vi "setRootDevice.vi"(8 "error in (no error)":errorcluster, 9 "Config in":refnum<class "IPropertyObject.lvclass">, 10 "Connection String in":string, 11 "IInstance in":refnum<class "IInstance.lvclass">) -> (0 "error out":errorcluster, 1 "Config out":refnum<class "IPropertyObject.lvclass">, 2 "Connection String out":string, 3 "IInstance out":refnum<class "IInstance.lvclass">)   [LabVIEW 2022 SP3, in "openDAQ.lvlib" / "IBaseObject.lvlib" / "IPropertyObject.lvlib" / "IComponent.lvlib" / "IFolder.lvlib" / "IDevice.lvlib" / "IInstance.lvlib" / "IInstance.lvclass"]
uses:
  <instrlib>/openDAQ/Public/Classes/IInstance/IInstance.lvclass
  C:/Program Files (x86)/National Instruments/LabVIEW 2022/instr.lib/openDAQ/Public/Classes/IBaseObject/IBaseObject.lvclass
  <instrlib>/openDAQ/Public/Classes/IPropertyObject/IPropertyObject.lvclass
  <instrlib>/openDAQ/Public/Classes/IBaseObject/IBaseObject.lvclass/IBaseObject.ctl
  <instrlib>/openDAQ/Public/Classes/IBaseObject/Accessor/Read reference.vi
  <instrlib>/openDAQ/Public/Classes/IBaseObject/Accessor/Write reference.vi
  <instrlib>/openDAQ/Public/Classes/daqCoreTypes/IString/IString.lvclass
  <instrlib>/openDAQ/Binaries/Windows/x86/copendaq32.dll
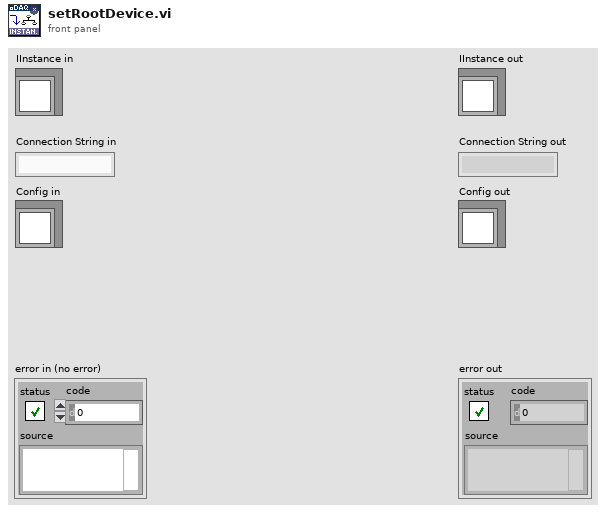
[diagram p1: front panel]
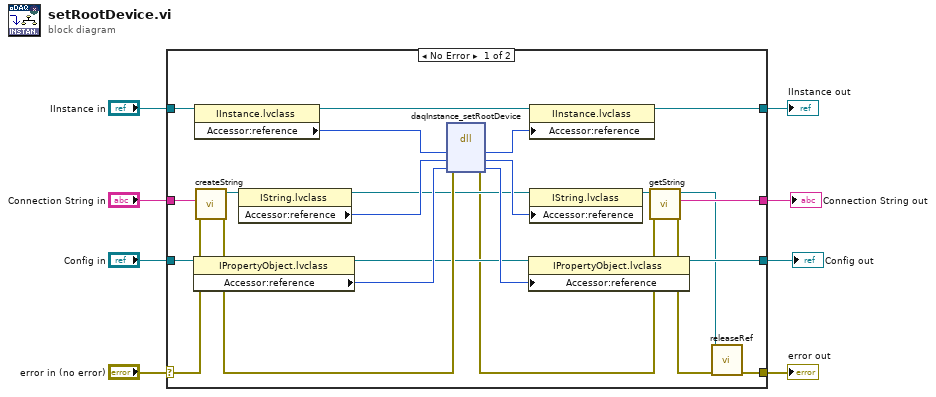
[diagram p0: block diagram]
diagram:
  n1 = case shown="No Error" "error in (no error)" {
    selector: "error in (no error)" -> [w24 w35]
    tunnel: [w10 w35] -> w7
    tunnel: [w29 w34] -> w5
    tunnel: "IInstance in" -> [w30 w34]
    tunnel: "Config in" -> [w27 w32]
    tunnel: "Connection String in" -> [w25 w33]
    tunnel: [w13 w33] -> w2
    tunnel: [w12 w32] -> w1
    frame No Error {
      n2 = property class="IPropertyObject.lvclass"(reference=w27) -> (reference out=w19:refnum<class "IPropertyObject.lvclass">, "Accessor:reference"=w20:i64)  [unwired: 1 in, 1 out]
      n3 = property class="IInstance.lvclass"(reference=w30) -> (reference out=w28:refnum<class "IInstance.lvclass">, "Accessor:reference"=w26:i64)  [unwired: 1 in, 1 out]
      n4 = call <instrlib>:"createString.vi"("error in (no error)"=w24, "String"=w25) -> ("error out"=w23:errorcluster, "IString out"=w22:refnum<class "IString.lvclass">)  [unwired: 8 in]
      n5 = property class="IString.lvclass"(reference=w22) -> (reference out=w16:refnum<class "IString.lvclass">, "Accessor:reference"=w21:i64)  [unwired: 1 in, 1 out]
      n6 = dll-call lib="C:/Program Files (x86)/National Instruments/LabVIEW 2022/instr.lib/openDAQ/Binaries/Windows/x86/copendaq*.*" fn="daqInstance_setRootDevice"(error in=w23, "instance"=w26, "connectionString"=w21, "config"=w20) -> (error out=w14:errorcluster, "instance"=w17:i64, "connectionString"=w18:i64, "config"=w31:i64)  [unwired: 3 in, 1 out]
      n7 = property class="IPropertyObject.lvclass"(reference=w19, "Accessor:reference"=w31) -> (reference out=w12:refnum<class "IPropertyObject.lvclass">)  [unwired: 1 in, 1 out]
      n8 = property class="IInstance.lvclass"(reference=w28, "Accessor:reference"=w17) -> (reference out=w29:refnum<class "IInstance.lvclass">)  [unwired: 1 in, 1 out]
      n9 = property class="IString.lvclass"(reference=w16, "Accessor:reference"=w18) -> (reference out=w15:refnum<class "IString.lvclass">)  [unwired: 1 in, 1 out]
      n10 = call <instrlib>:"getString.vi"("error in (no error)"=w14, "IString in"=w15) -> ("error out"=w11:errorcluster, "String out"=w13:string, "IString out"=w9:refnum<class "IString.lvclass">)  [unwired: 7 in]
      n11 = call-dynamic "releaseRef.vi"("error in (no error)"=w11, "IBaseObject in"=w9) -> ("error out"=w10:errorcluster)  [unwired: 9 in]
    }
    frame Error {
    }
  }
  "error out" <- w7
  "IInstance out" <- w5
  "Connection String out" <- w2
  "Config out" <- w1
